vi "CD Init_Prepare Async Data_BC to RT.vi"(8 "error in (no error)":errorcluster, 10 "Card Parameters (in)":T5, 11 "Channels In":T12[](array[typedef]) {"RTs"."Mode Codes"."param item refs" format="%.0x"; "RTs"."Mode Codes"."Timestamp Channel Data Reference" format="%.0x"; "RTs"."subAddresses"."param item refs" format="%.0x"; "RTs"."subAddresses"."Timestamp Channel Data Reference" format="%.0x"; "RTs"."Status Channel Data Reference" format="%.0x"; "RTs"."Command Channels Refs" format="%.0x"; "BC"."Acyclic Frames Trigger Channels Refs" format="%.0x"; "BC"."Command Channels Refs" format="%.0x"; "BC"."messages"."Timestamp Channel Data Reference" format="%.0x"; "BC"."messages"."Status Channel Data Refs" format="%.0x"; "BC"."messages"."param item refs" format="%.0x"; "BC"."messages"."param Block Data Refs"."Data Reference" format="%.0x"}) -> (0 "error out":errorcluster, 1 "param map (BC to RT)":T1, 2 "Raw Values (BC to RT)":T7, 3 "Map (BC to RT)":T9[](array[typedef]) {"Channel Data Reference" format="%.0x"})   [LabVIEW 2020, in "Ballard MIL-1553 Engine.lvlib"]
doc: "This VI creates a static association between NI-VS FIFO Channel Index and Physical Channel, Label Index, Parameter Index for Parameter Channel of a Tx Scheduled Label."
uses:
  Ballard MIL-1553 Engine.lvlib
  Shared/Controls and Global/RT Channel.ctl
  Shared/Controls and Global/RT BC.ctl
  <vilib>/NI VeriStand/Custom Device API/Custom Device Item Ref.ctl
  Shared/Controls and Global/RT Message.ctl
  Shared/Controls and Global/RT messageType.ctl
  Shared/Controls and Global/RT CWD1.ctl
  Shared/Controls and Global/RT CWD2.ctl
  <vilib>/NI VeriStand/Custom Device API/Data Reference.ctl
  <vilib>/NI VeriStand/Custom Device API/Block Data Reference.ctl
  Shared/EncodeDecode/_typedefs/parameter_config_type.ctl
  Shared/EncodeDecode/_typedefs/parameter_config_type_type.ctl
  Shared/EncodeDecode/_typedefs/parameter_config_encoding_type.ctl
  Shared/Controls and Global/RT Remote Terminal.ctl
  Shared/Controls and Global/RT Remote Terminal_rtMode.ctl
  Shared/Controls and Global/RT Remote Terminal_RT subAddress.ctl
  Shared/Controls and Global/RT Remote Terminal_RT direction.ctl
  Shared/Controls and Global/RT Remote Terminal_RT Mode Code.ctl
  Controls/RT Async_Map BC2RT.ctl
  Controls/RT Async_Map_Type.ctl
  Controls/RT Async_Raw Values.ctl
  Controls/RT Async_Raw Values to Messages Index_Association.ctl
  Controls/Card Parameters.ctl
  Shared/Controls and Global/Initialization Method.ctl
  Controls/Asynchronous - Parameter map_type.ctl
  <vilib>/NI VeriStand/Custom Device API/Custom Device API.lvlib
  <instrlib>/BTI1553Lib/BTI1553LV.lvlib
  Shared/Ballard 1553 Shared.lvlib
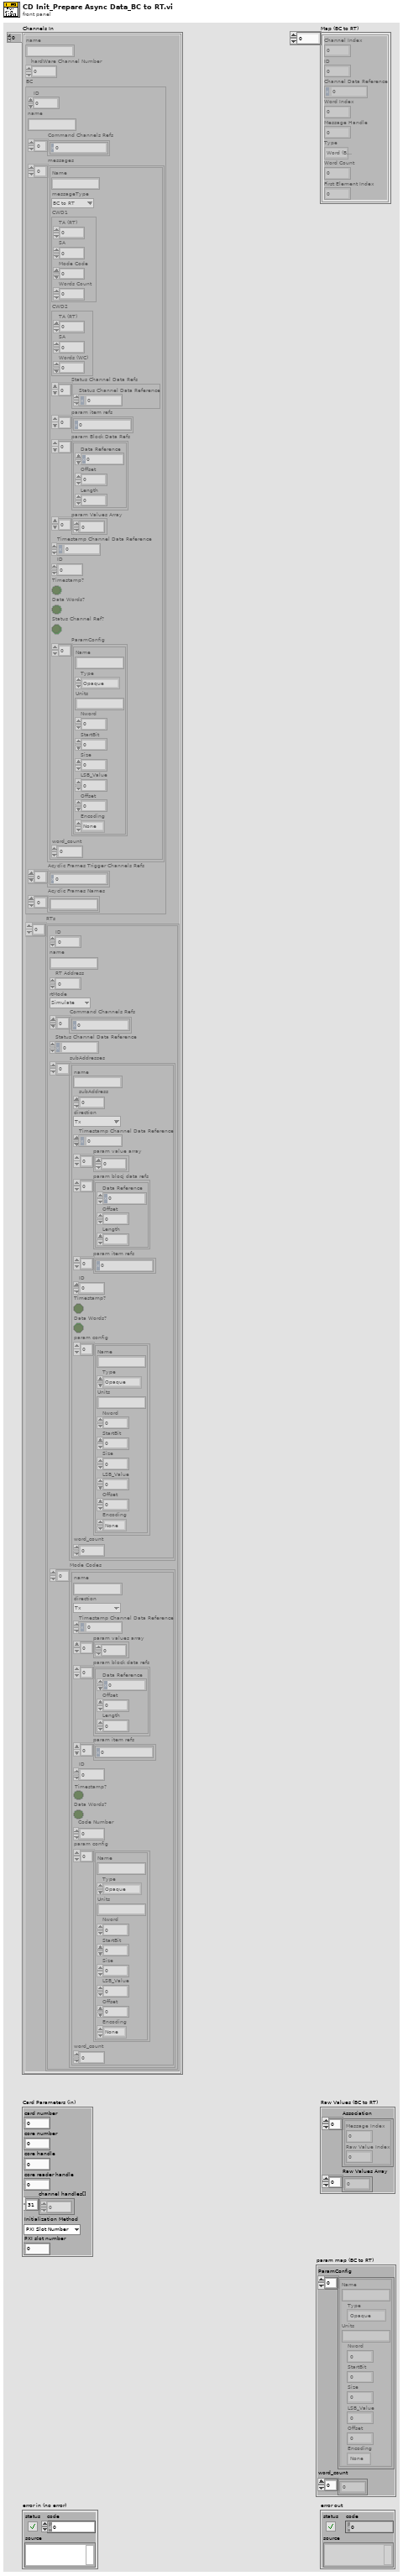
[diagram p1: front panel]
types:
  T1 = typedef "Ballard MIL-1553 Engine.lvlib/Asynchronous - Parameter map_type.ctl" = cluster{"ParamConfig":T2[], "word_count":u8[]}
  T2 = typedef "parameter_config_type.ctl" = cluster{"Name":string, "Type":T3, "Units":string, "Nword":i32, "StartBit":i32, "Size":i32, "LSB_Value":i32, "Offset":i32, "Encoding":T4}
  T3 = typedef "parameter_config_type_type.ctl" = enum16{"Opaque", "Enum", "Float", "Integer", "Bcd", "Bool"}
  T4 = typedef "parameter_config_encoding_type.ctl" = enum16{"None", "2-complement", "Unsigned"}
  T5 = typedef "Ballard MIL-1553 Engine.lvlib/Card Parameters.ctl" = cluster{"card number":i32, "core number":i32, "core handle":u64, "core reader handle":u64, "channel handles[]":u64[], "Initialization Method":T6, "PXI slot number":i32}
  T6 = typedef "Ballard 1553 Shared.lvlib/Initialization Method.ctl" = enum16{"PXI Slot Number", "Card Number"}
  T7 = typedef "Ballard MIL-1553 Engine.lvlib/RT Async_Raw Values.ctl" = cluster{"Association":T8[], "Raw Values Array":u16[]}
  T8 = typedef "Ballard MIL-1553 Engine.lvlib/RT Async_Raw Values to Messages Index_Association.ctl" = cluster{"Message Index":i32, "Raw Value Index":i32}
  T9 = typedef "Ballard MIL-1553 Engine.lvlib/RT Async_Map BC2RT.ctl" = cluster{"Channel Index":i32, "ID":i32, "Channel Data Reference":T10, "Word Index":i32, "Message Handle":u64, "Type":T11, "Word Count":i32, "First Element Index":i32}
  T10 = typedef "Custom Device API.lvlib/Data Reference.ctl" = i32
  T11 = typedef "Ballard MIL-1553 Engine.lvlib/RT Async_Map_Type.ctl" = enum16{"Word (BC to RT)", "Word (MC (Rx))", "Acyclic Message Trigger", "Word (RT to ..)", "Word (RT to RT)", "Word (MC (Tx))", "RT Status", "BC Commands", "RT Commands"}
  T12 = typedef "Ballard 1553 Shared.lvlib/RT Channel.ctl" = cluster{"name":string, "hardWare Channel Number":u16, "BC":T13, "RTs":T20[]}
  T13 = typedef "Ballard 1553 Shared.lvlib/RT BC.ctl" = cluster{"ID":i32, "name":string, "Command Channels Refs":T14[], "messages":T15[], "Acyclic Frames Trigger Channels Refs":T14[], "Acyclic Frames Names":string[]}
  T14 = typedef "Custom Device API.lvlib/Custom Device Item Ref.ctl" = u64
  T15 = typedef "Ballard 1553 Shared.lvlib/RT Message.ctl" = cluster{"Name":string, "messageType":T16, "CWD1":T17, "CWD2":T18, "Status Channel Data Refs":T10[], "param item refs":T14[], "param Block Data Refs":T19[], "param Values Array":u16[], "Timestamp Channel Data Reference":T10, "ID":i32, "Timestamp?":bool, "Data Words?":bool, "Status Channel Ref?":bool, "ParamConfig":T2[], "word_count":u8}
  T16 = typedef "Ballard 1553 Shared.lvlib/RT messageType.ctl" = enum16{"BC to RT", "RT to BC", "RT to RT", "MC (Rx)", "MC (Tx)"}
  T17 = typedef "Ballard 1553 Shared.lvlib/RT CWD1.ctl" = cluster{"TA (RT)":i8, "SA":i8, "Mode Code":i8, "Words Count":i8}
  T18 = typedef "Ballard 1553 Shared.lvlib/RT CWD2.ctl" = cluster{"TA (RT)":i8, "SA":i8, "Words (WC)":i8}
  T19 = typedef "Custom Device API.lvlib/Block Data Reference.ctl" = cluster{"Data Reference":T10, "Offset":u64, "Length":u64}
  T20 = typedef "Ballard 1553 Shared.lvlib/RT Remote Terminal.ctl" = cluster{"ID":i32, "name":string, "RT Address":i32, "rtMode":T21, "Command Channels Refs":T14[], "Status Channel Data Reference":T10, "subAddresses":T22[], "Mode Codes":T24[]}
  T21 = typedef "Ballard 1553 Shared.lvlib/RT Remote Terminal_rtMode.ctl" = enum16{"Simulate", "Monitor", "Disable"}
  T22 = typedef "Ballard 1553 Shared.lvlib/RT Remote Terminal_RT subAddress.ctl" = cluster{"name":string, "subAddress":i8, "direction":T23, "Timestamp Channel Data Reference":T10, "param value array":u16[], "param blocj data refs":T19[], "param item refs":T14[], "ID":i32, "Timestamp?":bool, "Data Words?":bool, "param config":T2[], "word_count":u8}
  T23 = typedef "Ballard 1553 Shared.lvlib/RT Remote Terminal_RT direction.ctl" = enum16{"Tx", "Rx"}
  T24 = typedef "Ballard 1553 Shared.lvlib/RT Remote Terminal_RT Mode Code.ctl" = cluster{"name":string, "direction":T23, "Timestamp Channel Data Reference":T10, "param values array":u16[], "param block data refs":T19[], "param item refs":T14[], "ID":i32, "Timestamp?":bool, "Data Words?":bool, "Code Number":i32, "param config":T2[], "word_count":u8}
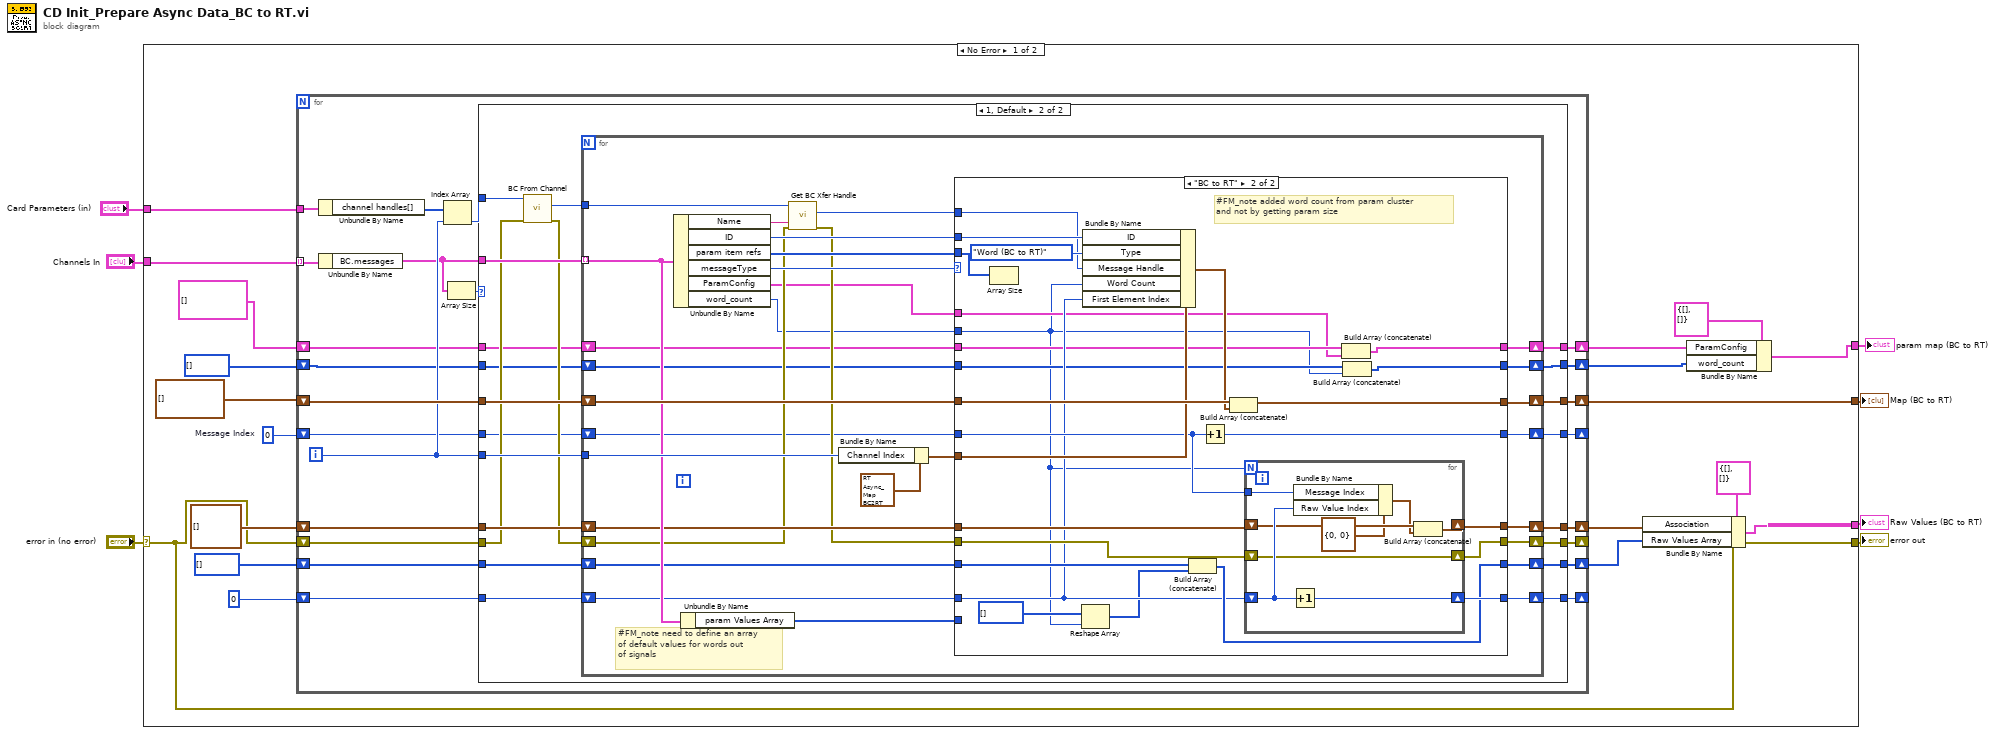
[diagram p0: block diagram]
diagram:
  n1 = case shown="No Error" "error in (no error)" {
    selector: "error in (no error)" -> [w16 w151]
    tunnel: [w16 w151] -> w6
    tunnel: "Channels In" -> [w26 _]
    tunnel: [w24 _] -> w4
    tunnel: [w20 _] -> w3
    tunnel: "Card Parameters (in)" -> [w17 _]
    tunnel: [w8 _] -> w1
    frame No Error {
      w15 = 0  # Message Index
      n2 = for {
        tunnel: w26 -> [w49] mode=indexing
        shift-right: [w47] -> w24
        shift-left: T9[] [] -> [w48]
        shift-right: [w45] -> w21
        shift-left: T8[] [] -> [w46]
        shift-right: [w41] -> w14
        shift-left: u16[] [] -> [w44]
        shift-right: [w42] -> _
        shift-left: 0 -> [w43]
        tunnel: w17 -> [w40]
        shift-right: [w37] -> _
        shift-left: w16 -> [w35]
        shift-right: [w33] -> _
        shift-left: w15 -> [w34]
        shift-right: [w27] -> w9
        shift-left: u8[] [] ("word_count") -> [w29]
        shift-right: [w28] -> w10
        shift-left: T2[] [] ("ParamConfig") -> [w30]
        i -> [w38]
        n3 = Unbundle By Name(w40) -> ("channel handles[]"=w39:u64[])
        n4 = Unbundle By Name(w49) -> ("BC.messages"=w31:T15[])
        n5 = Index Array(array=w39, index=w38) -> (element=w36:u64)
        n6 = Array Size(array=w31) -> (size(s)=w32:i32)
        n7 = case shown="1, Default" w32 {
          tunnel: w31 -> [_ w78]
          tunnel: w48 -> [w57 w77]
          tunnel: [w57 w76] -> w47
          tunnel: w46 -> [w55 w75]
          tunnel: [w55 w74] -> w45
          tunnel: w44 -> [w53 w73]
          tunnel: w43 -> [w52 w72]
          tunnel: [w52 w71] -> w42
          tunnel: [w53 w70] -> w41
          tunnel: w38 -> [_ w69]
          tunnel: [w54 w68] -> w37
          tunnel: w36 -> [_ w67]
          tunnel: w35 -> [w54 w66]
          tunnel: w34 -> [w56 w63]
          tunnel: [w56 w62] -> w33
          tunnel: w30 -> [w51 w61]
          tunnel: w29 -> [w50 w60]
          tunnel: [w51 w59] -> w28
          tunnel: [w50 w58] -> w27
          frame 0 {
          }
          frame 1, Default {
            n8 = call <instrlib>:"BC From Channel.vi"("error in (no error)"=w66, "channel handle in"=w67) -> ("error out"=w65:errorcluster, "bus controller handle out"=w64:u64)  [unwired: 7 in, 1 out]
            n9 = for {
              tunnel: w78 -> [w102] mode=indexing
              shift-right: [w87] -> w76
              shift-left: w77 -> [w106]
              tunnel: w69 -> [w107]
              shift-right: [w103] -> w74
              shift-left: w75 -> [w98]
              shift-right: [w101] -> w70
              shift-left: w73 -> [w97]
              shift-right: [w100] -> w71
              shift-left: w72 -> [w99]
              tunnel: w64 -> [w93]
              shift-right: [w89] -> w68
              shift-left: w65 -> [w91]
              shift-right: [w85] -> w62
              shift-left: w63 -> [w86]
              shift-right: [w79] -> w58
              shift-left: w60 -> [w83]
              shift-right: [w80] -> w59
              shift-left: w61 -> [w84]
              # "#FM_note need to define an array\nof default values for words out \nof signals"
              n10 = Unbundle By Name(w102) -> ("Name"=w92:string, "ID"=w94:i32, "param item refs"=w104:T14[], "messageType"=w95:T16, "ParamConfig"=w82:T2[], "word_count"=w81:u8)
              n11 = Unbundle By Name(w102) -> ("param Values Array"=w96:u16[])
              n12 = call <instrlib>:"Get BC Xfer Handle.vi"("error in (no error)"=w91, "bc transfer name"=w92, "bus controller handle in"=w93) -> ("error out"=w90:errorcluster, "bc transfer handle out"=w88:u64)  [unwired: 6 in, 1 out]
              n13 = Bundle By Name(cluster=T9 {"Channel Index"=0, "ID"=-1, "Channel Data Reference"=0, "Word Index"=0, "Message Handle"=0, "Type"=enum."Word (BC to RT)", "Word Count"=0, "First Element Index"=0} ("Association"), "Channel Index"=w107) -> (w105:T9)
              n14 = case shown="\"BC to RT\"" w95 {
                tunnel: w106 -> [w112 w132]
                tunnel: [w112 w131] -> w87
                tunnel: w105 -> [_ w129]
                tunnel: w104 -> [_ w126]
                tunnel: [w116 w142] -> w103
                tunnel: [w115 w138] -> w101
                tunnel: [w114 w141] -> w100
                tunnel: w99 -> [w114 w125]
                tunnel: w98 -> [w116 w140]
                tunnel: w97 -> [w115 w139]
                tunnel: w96 -> [_ _]
                tunnel: w88 -> [_ w133]
                tunnel: w94 -> [_ w134]
                tunnel: w90 -> [w113 w137]
                tunnel: [w113 w136] -> w89
                tunnel: w86 -> [w111 w127]
                tunnel: [w111 w128] -> w85
                tunnel: w84 -> [w110 w124]
                tunnel: w83 -> [w109 w121]
                tunnel: w82 -> [_ w123]
                tunnel: w81 -> [_ w118]
                tunnel: [w110 w122] -> w80
                tunnel: [w109 w120] -> w79
                frame Default {
                  # "We don't care."
                }
                frame "BC to RT" {
                  # "#FM_note added word count from param cluster\nand not by getting param size"
                  n15 = Array Size(array=w126) -> ()  [unwired: 1 out]
                  n16 = Reshape Array(u16[] [] ("param value array"), w118) -> (w117:u16[])
                  n17 = Bundle By Name(cluster=w129, "ID"=w134, "Type"=RT_Async_Map_Type."Word (BC to RT)", "Message Handle"=w133, "Word Count"=w118, "First Element Index"=w125) -> (w130:T9)
                  n18 = Build Array (concatenate)(w139, w117) -> (w138:u16[])
                  n19 = Increment(x=w127) -> (x+1=w128:i32)
                  n20 = Build Array (concatenate)(w132, w130) -> (w131:T9[])
                  n21 = for {
                    N: w118 -> [_]
                    shift-right: [w149] -> w141
                    shift-left: w125 -> [w148]
                    shift-right: [w146] -> w136
                    shift-left: w137 -> [w146]
                    tunnel: w127 -> [w143]
                    shift-right: [w150] -> w142
                    shift-left: w140 -> [w147]
                    n22 = Increment(x=w148) -> (x+1=w149:i32)
                    n23 = Bundle By Name(cluster=T8 {"Message Index"=0, "Raw Value Index"=0} ("Cluster"), "Message Index"=w143, "Raw Value Index"=w148) -> (w145:T8)
                    n24 = Build Array (concatenate)(w147, w145) -> (w150:T8[])
                  }
                  n25 = Build Array (concatenate)(w124, w123) -> (w122:T2[])
                  n26 = Build Array (concatenate)(w121, w118) -> (w120:u8[])
                }
              }
            }
          }
        }
      }
      n27 = Bundle By Name(cluster=T7 {"Association"=[], "Raw Values Array"=[]} ("Raw Values"), "Association"=w21, "Raw Values Array"=w14) -> (w20:T7)
      n28 = Bundle By Name(cluster=T1 {"ParamConfig"=[], "word_count"=[]}, "ParamConfig"=w10, "word_count"=w9) -> (w8:T1)
    }
    frame Error {
    }
  }
  "error out" <- w6
  "Map (BC to RT)" <- w4
  "Raw Values (BC to RT)" <- w3
  "param map (BC to RT)" <- w1
